vi "TDMSViewerStart.vi"(0 "TDMSFilePath":path) -> ()   [LabVIEW 2025, in "ZE_Recorder.lvlib"]
doc: "ZE_Recorder.lvlib:TDMSViewerStart.vi\n----------------------------------------------\nOpens a filedialog with the TDMSFilePath as Startvalue and TDMS as Filepattern. Opens the TDMS File Viewer with the choosen File. If the dialog is canceled, no Viewer is opened.\n\nInputs:\n---------------------\n- TDMSFilePath : Path; \n\nOutputs:\n---------------------\n\n\n----------------------------------------------\n13.08.2020, wer\nZühlke Engineering AG\nCH-8952 Schlieren\nwww.zuehlke.com"
uses:
  ZE_Recorder.lvlib
  <vilib>/Utility/TDMS File Viewer/NI_TDMS File Viewer.lvlib
panel:
  out "error IO":errorcluster
  # "Connector Pane"
  # "Locals"
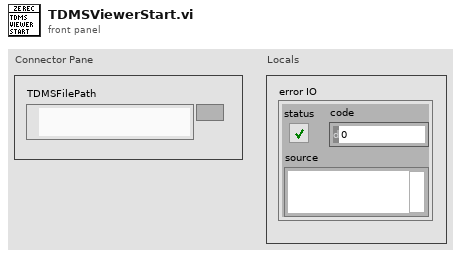
[diagram p1: front panel]
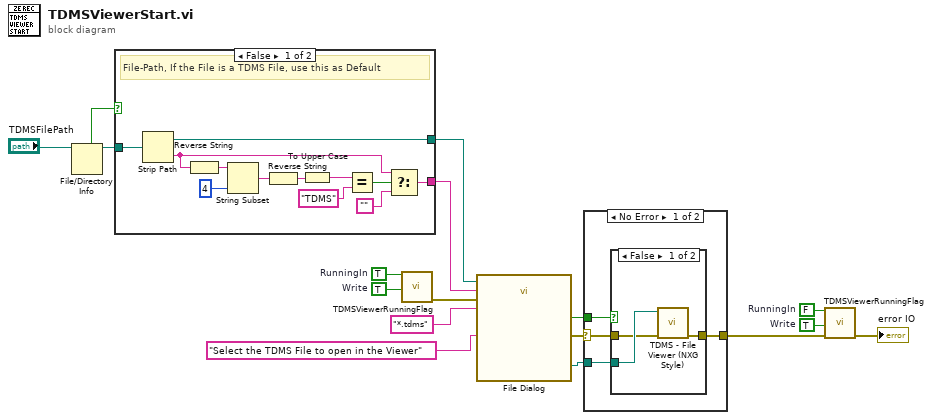
[diagram p0: block diagram]
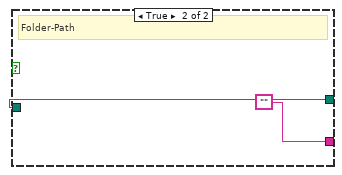
[diagram p2: hidden frame]
diagram:
  w9 = TRUE  # Write
  w8 = TRUE  # RunningIn
  w10 = TRUE  # Write
  w11 = FALSE  # RunningIn
  n1 = File/Directory Info(path="TDMSFilePath") -> (directory=w4:bool)  [unwired: 1 in, 6 out]
  n2 = case shown="False" w4 {
    tunnel: "TDMSFilePath" -> [w28 w30]
    tunnel: [w27 w30] -> w2
    tunnel: [w23 ""] -> w1
    frame False {
      # "File-Path, If the File is a TDMS File, use this as Default"
      n3 = Strip Path(path=w28) -> (stripped path=w27:path, name=w21:string)
      n4 = Reverse String(1:w21) -> (0:w20:string)
      n5 = String Subset(string=w20, length (rest)=4 ("length (rest)")) -> (substring=w18:string)  [unwired: 1 in]
      n6 = Reverse String(1:w18) -> (0:w17:string)
      n7 = To Upper Case(1:w17) -> (0:w25:string)
      n8 = Equal?(x=w25, y="TDMS" ("x")) -> (x = y?=w24:bool)
      n9 = Select(t=w21, s=w24, f="") -> (s? t:f=w23:string)
    }
    frame True {
      # "Folder-Path"
    }
  }
  n10 = call "TDMSViewerRunningFlag.vi"("RunningIn"=w8, "Write"=w9) -> ("error out"=w7:errorcluster)  [unwired: 12 in, 1 out]
  n11 = call "File Dialog"("start path"=w2, "prompt"="Select the TDMS File to open in the Viewer", "default name"=w1, "error in"=w7, "pattern (all files)"="*.tdms") -> ("selected path"=w16:path, "cancelled"=w14:bool, "error out"=w15:errorcluster)  [unwired: 7 in, 1 out]
  n12 = case shown="No Error" w15 {
    selector: w15 -> [w32 w39]
    tunnel: w16 -> [w34 _]
    tunnel: w14 -> [w33 _]
    tunnel: [w31 w39] -> w12
    frame No Error {
      n13 = case shown="False" w33 {
        tunnel: w34 -> [w37 _]
        tunnel: w32 -> [w36 w38]
        tunnel: [w35 w38] -> w31
        frame False {
          n14 = call <vilib>:"TDMS - File Viewer (NXG Style).vi"("error in"=w36, "file in"=w37) -> ("error out"=w35:errorcluster)  [unwired: 8 in, 1 out]
        }
        frame True {
          # "Canceled"
        }
      }
    }
    frame Error {
    }
  }
  n15 = call "TDMSViewerRunningFlag.vi"("RunningIn"=w11, "Write"=w10, "error in"=w12) -> ("error out"=→"error IO":errorcluster)  [unwired: 11 in, 1 out]
